vi "Empty Ring StringsAndValues.vi"(8 "error in (no error)":errorcluster, 11 "Ring in":refnum<vi>) -> (0 "error out":errorcluster, 3 "Ring out":refnum<vi>)   [LabVIEW 2019, in "Control Experiment.lvclass"]
uses:
  Control Experiment.lvclass
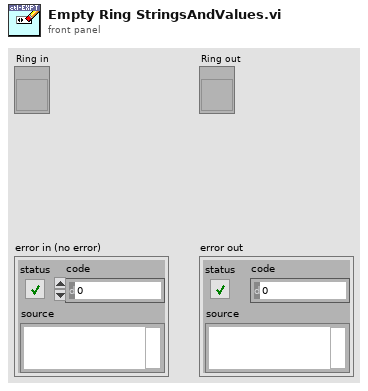
[diagram p1: front panel]
types:
  T1 = typedef "LVStringsAndValuesArrayTypeDef.ctl" = cluster{"String":string, "Value":ext}[]
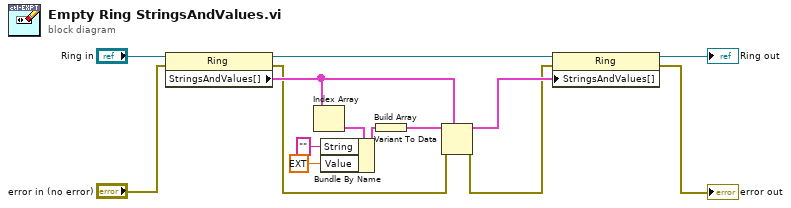
[diagram p0: block diagram]
diagram:
  n1 = property class="Ring"(reference="Ring in", error in="error in (no error)") -> (reference out=w11:refnum<vi>, error out=w1:errorcluster, "StringsAndValues[]"=w6:T1)
  n2 = Index Array(array=w6) -> (element=w7:cluster{"String":string, "Value":ext})  [unwired: 1 in]
  n3 = Bundle By Name(cluster=w7, "String"="", "Value"=ext 0.0) -> (w10:cluster{"String":string, "Value":ext})
  n4 = Build Array(w10) -> (w5:cluster{"String":string, "Value":ext}[])
  n5 = Variant To Data(error in=w1, type=w6, Variant=w5) -> (data=w4:T1, error out=w3:errorcluster)
  n6 = property class="Ring"(reference=w11, error in=w3, "StringsAndValues[]"=w4) -> (reference out=→"Ring out":refnum<vi>, error out=→"error out":errorcluster)
